vi "test_F5730.vi"() -> ()   [LabVIEW 2020]
uses:
  external libraries/Fluke 5XXX Series Multicalibrator/Fluke 5XXX Series Multicalibrators.lvlib
panel:
  in  "Output Value(s) (0 - Amplitude)":u32(ring)=3 items=["Amplitude", "Volts dc or update volts ac", "Volts ac dBm update", "Volts ac or volts dc with 0 Hz", "Volts ac in dBm", "Current dc or update current ac", "Current ac", "Update frequency", "Resistance", "Capacitance", "Temperature (Celsius)", "Temperature (Fahrenheit)", "Power dc or update power ac", "Power ac", "Dual volts dc or update dual ac", "Dual volts ac in volts", "Power ac in dBm update", "Power ac in dBm", "Dual volts ac in dBm update", "Dual volts ac in dBm"]
  in  "Stop":bool
  out "appended array":errorcluster[](array[cluster])
  in  "VISA resource name":refnum<visa-resource-name>
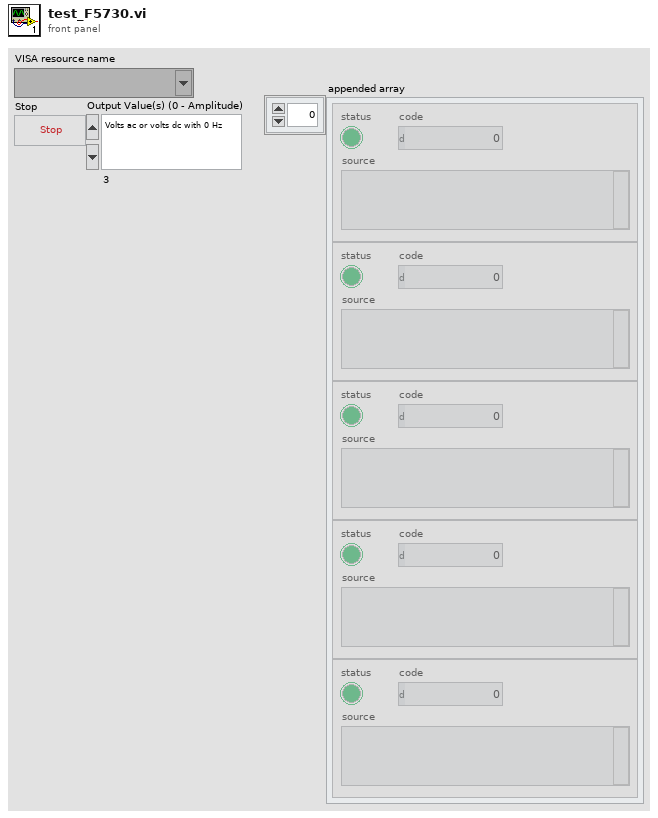
[diagram p1: front panel]
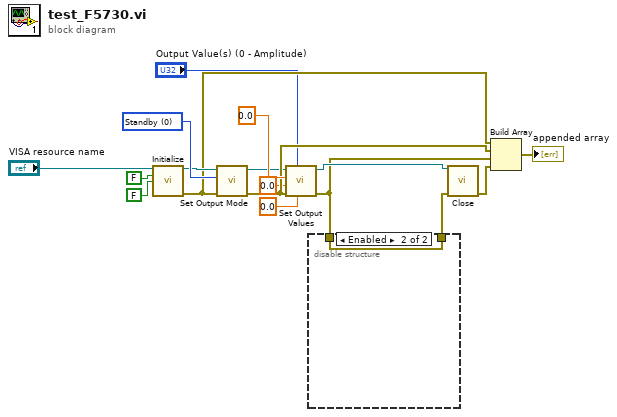
[diagram p0: block diagram]
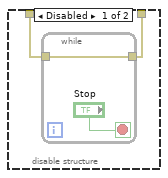
[diagram p2: hidden frame]
diagram:
  w11 = u32 0 items=["Standby", "Operate"] ("Output Mode (0: Standby)")
  n1 = call "Initialize.vi"("VISA resource name"="VISA resource name", "ID Query (T: Check)"=FALSE, "Reset (T: Reset)"=FALSE) -> ("VISA resource name out"=w10:refnum<visa-resource-name>, "error out"=w9:errorcluster)  [unwired: 11 in]
  n2 = call "Set Output Mode.vi"("error in (no error)"=w9, "Output Mode (0: Standby)"=w11, "VISA resource name"=w10) -> ("error out"=w7:errorcluster, "VISA resource name out"=w6:refnum<visa-resource-name>)  [unwired: 7 in]
  n3 = call "Set Output Values.vi"("Fundamental Frequency (0.0 Hz)"=0.0, "Output Value(s) (0 - Amplitude)"="Output Value(s) (0 - Amplitude)", "error in (no error)"=w7, "Secondary Value (0.0)"=0.0, "Primary Value (0.0)"=0.0, "VISA resource name"=w6) -> ("error out"=w3:errorcluster, "VISA resource name out"=w5:refnum<visa-resource-name>)  [unwired: 4 in]
  n4 = disable-structure shown="Enabled" {
    disable-tunnel: [w19 w22] -> w12
    disable-tunnel: w3 -> [w18 w22]
    frame Disabled {
      n5 = while {
        tunnel: [w20] -> w19
        tunnel: w18 -> [w20]
        stop <- "Stop" stop-if-true
      }
    }
    frame Enabled {
    }
  }
  n6 = call "Close.vi"("VISA resource name"=w5, "error in (no error)"=w12) -> ("error out"=w14:errorcluster)  [unwired: 13 in]
  n7 = Build Array(w9, w7, w3, w14) -> (→"appended array":errorcluster[])
